vi "FlatToRichhwval_ExportRequest.vi"(5 "OutputClusterType":T1, 11 "InputCluster":T2) -> (3 "OutputCluster":T1)   [LabVIEW 2025, in "Automotive-Vision-OOBService_client.lvlib"]
uses:
  Automotive-Vision-OOBService_client.lvlib
  hwval_ExportRequest_Flat.ctl
  hwval_ExportRequest.ctl
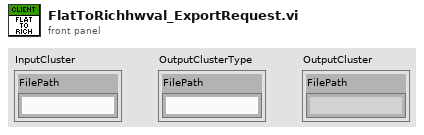
[diagram p1: front panel]
types:
  T1 = typedef "Automotive-Vision-OOBService_client.lvlib/hwval_ExportRequest.ctl" = cluster{"FilePath":string}
  T2 = typedef "Automotive-Vision-OOBService_client.lvlib/hwval_ExportRequest_Flat.ctl" = cluster{"FilePath":string}
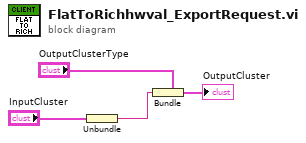
[diagram p0: block diagram]
diagram:
  n1 = Unbundle "Unbundle"("InputCluster") -> ("FilePath"=w1:string)
  n2 = Bundle "Bundle"(cluster="OutputClusterType", "FilePath"=w1) -> (→"OutputCluster":T1)
